vi "PRUEBA_A_PWM.vi"() -> ()   [LabVIEW 2025]
panel:
  out "DC":u8
  in  "Pin":u8=4 min=4 max=40
  out "Analog read":u16
  in  "stop":bool
  in  "VISA resource name":refnum<visa-resource-name>
  out "error out":errorcluster
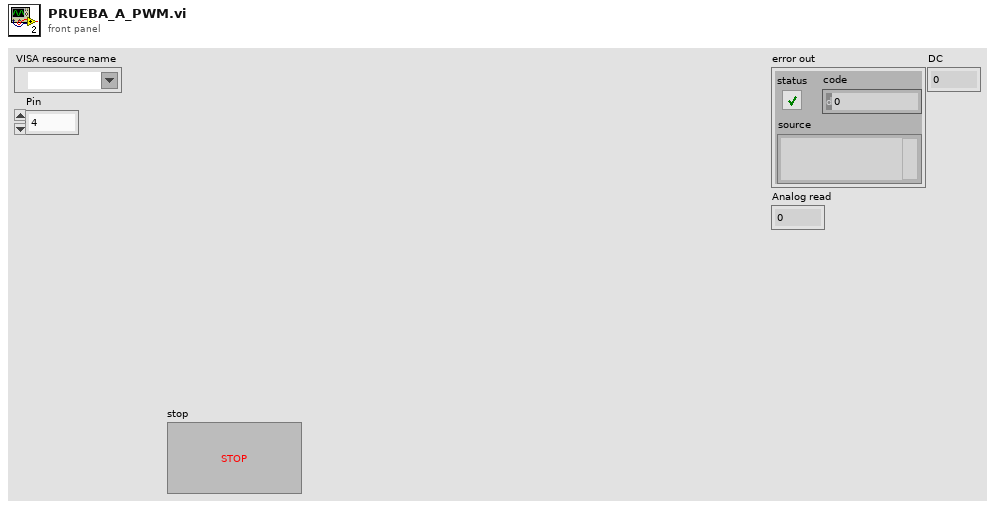
[diagram p1: front panel]
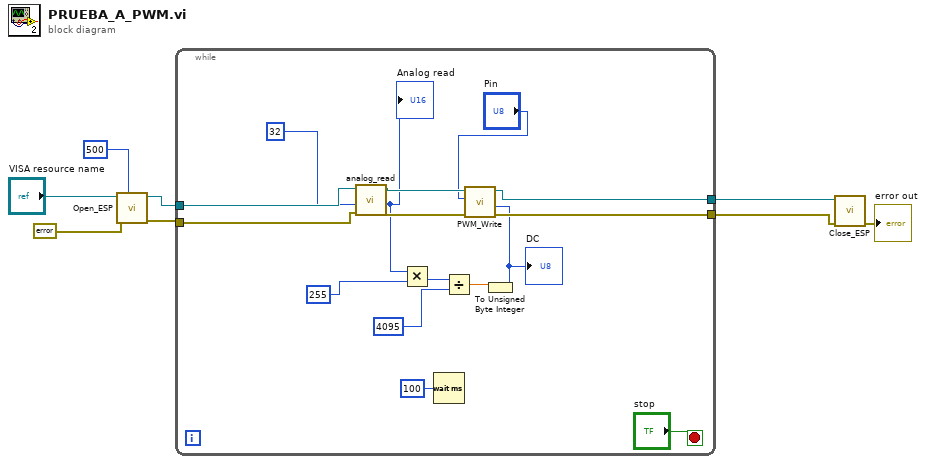
[diagram p0: block diagram]
diagram:
  n1 = call "Open_ESP.vi"("timeout (10sec)"=u32 500, "error in (no error)"=errorcluster {"status"=FALSE, "code"=0, "source"=""}, "VISA resource name"="VISA resource name") -> ("error out"=w7:errorcluster, "VISA resource name out"=w8:refnum<visa-resource-name>)  [unwired: 7 in]
  n2 = while {
    tunnel: w8 -> [w22]
    tunnel: w7 -> [w23]
    tunnel: [w18] -> w2
    tunnel: [w17] -> w1
    stop <- "stop" stop-if-true
    n3 = call "analog_read.vi"("error in (no error)"=w23, "Pin"=u8 32, "VISA resource name"=w22) -> ("error out"=w16:errorcluster, "Analog read"=w10:u16, "VISA resource name out"=w19:refnum<visa-resource-name>)  [unwired: 6 in]
    "Analog read" <- w10
    n4 = Multiply(x=w10, y=255) -> (x*y=w13:i32)
    n5 = Wait (ms)(milliseconds to wait=u32 100) -> ()  [unwired: 1 out]
    n6 = Divide(x=w13, y=4095) -> (x/y=w11:dbl)
    n7 = To Unsigned Byte Integer(number=w11) -> (unsigned 8bit integer=w9:u8)
    "DC" <- w9
    n8 = call "PWM_Write.vi"("error in (no error)"=w16, "DC"=w9, "Pin"="Pin", "VISA resource name"=w19) -> ("error out"=w17:errorcluster, "VISA resource name out"=w18:refnum<visa-resource-name>)  [unwired: 6 in]
  }
  n9 = call "Close_ESP.vi"("error in (no error)"=w1, "VISA resource name"=w2) -> ("error out"=→"error out":errorcluster)  [unwired: 9 in]
